vi "Main.vi"() -> ()   [LabVIEW 2021]
doc: "The myRIO Project template acquires acceleration data from the onboard accelerometer and displays the changes of acceleration values in a waveform chart."
uses:
  <vilib>/myRIO/Instrument Drivers/Onboard IO/AI/typedefs/AI Reference.ctl
  <vilib>/myRIO/Common/Instrument Driver Framework/Utilities/typedefs/myRIO Generic Hardware Reference.ctl
  <vilib>/myRIO/Common/Instrument Driver Framework/Utilities/typedefs/Hardware Version Enum.ctl
  <vilib>/myRIO/Common/Instrument Driver Framework/Utilities/typedefs/myRIO v1.0 Reference.ctl
  <vilib>/myRIO/Common/Instrument Driver Framework/Utilities/typedefs/Generic FPGA Reference.ctl
  <vilib>/myRIO/Common/Instrument Driver Framework/myRIO v1.0/AI/typedefs/AI Channels List.ctl
  <vilib>/myRIO/Common/Instrument Driver Framework/myRIO v1.0/AI/typedefs/AI Channels Enum.ctl
  <vilib>/myRIO/Common/Instrument Driver Framework/Utilities/typedefs/Analog Scaling Constants List.ctl
  <vilib>/myRIO/Common/Instrument Driver Framework/Utilities/typedefs/Analog Scaling Constants.ctl
  <vilib>/userDefined/High Color/nirio_resource_hc.ctl
  <vilib>/myRIO/Instrument Drivers/Onboard IO/DIO/typedefs/DIO Reference.ctl
  <vilib>/myRIO/Common/Instrument Driver Framework/myRIO v1.0/DIO/typedefs/DIO Channels List.ctl
  <vilib>/myRIO/Common/Instrument Driver Framework/myRIO v1.0/DIO/typedefs/DIO Channels Enum.ctl
  <vilib>/myRIO/Common/Instrument Driver Framework/myRIO v1.0/AI/vis/myRIO v1.1 Open AI.vi
  <vilib>/myRIO/Common/Instrument Driver Framework/myRIO v1.0/DIO/vis/myRIO v1.1 Open DIO.vi
  <vilib>/myRIO/Common/Instrument Driver Framework/Utilities/vis/Validate Channels.vi
  <vilib>/myRIO/Common/Instrument Driver Framework/myRIO v1.0/AI/vis/myRIO v1.0 Reserve AI.vi
  <vilib>/myRIO/Common/Instrument Driver Framework/myRIO v1.0/DIO/vis/myRIO v1.0 Reserve DIO.vi
  <vilib>/myRIO/Common/Instrument Driver Framework/myRIO v1.0/AI/vis/myRIO v1.0 Close AI.vi
  <vilib>/myRIO/Common/Instrument Driver Framework/myRIO v1.0/DIO/vis/myRIO v1.0 Close DIO.vi
  <vilib>/myRIO/Common/Instrument Driver Framework/myRIO v1.0/AI/vis/myRIO v1.0 Build MUX Configuration AI.vi
  <vilib>/myRIO/Common/Instrument Driver Framework/myRIO v1.0/Resource Manager/vis/myRIO v1.0 Reserve Channel List.vi
  <vilib>/myRIO/Common/Instrument Driver Framework/myRIO v1.0/DIO/vis/myRIO v1.0 Build MUX Configuration DIO.vi
  <vilib>/myRIO/Common/Instrument Driver Framework/myRIO v1.0/AI/vis/myRIO v1.0 Unreserve AI.vi
  <vilib>/myRIO/Common/Instrument Driver Framework/myRIO v1.0/DIO/vis/myRIO v1.0 Unreserve DIO.vi
  <vilib>/myRIO/Common/Instrument Driver Framework/myRIO v1.0/Resource Manager/vis/myRIO v1.0 Reserve Channel.vi
  <vilib>/myRIO/Common/Instrument Driver Framework/myRIO v1.0/Resource Manager/vis/myRIO v1.0 Unreserve Channel.vi
  <vilib>/myRIO/Common/Instrument Driver Framework/myRIO v1.0/Resource Manager/vis/myRIO v1.0 Create Configuration List.vi
  <vilib>/myRIO/Common/Instrument Driver Framework/myRIO v1.0/Resource Manager/vis/myRIO v1.0 Unreserve Channel List.vi
  <vilib>/myRIO/Common/Instrument Driver Framework/myRIO v1.0/Resource Manager/vis/myRIO v1.0 Build Mutex Name.vi
  <vilib>/Utility/VariantDataType/GetNumericInfo.vi
  <vilib>/Utility/error.llb/Error Cluster From Error Code.vi
  <vilib>/myRIO/Common/Instrument Driver Framework/myRIO v1.0/myRIO v1.1 Open.vi
  <vilib>/myRIO/Common/Instrument Driver Framework/Utilities/vis/IO Manager.vi
  <vilib>/myRIO/Common/Instrument Driver Framework/Utilities/vis/Configuration Manager.vi
  <vilib>/myRIO/Common/Instrument Driver Framework/myRIO v1.0/Resource Manager/vis/myRIO v1.0 Configure IO.vi
  <vilib>/myRIO/Common/Instrument Driver Framework/myRIO v1.0/myRIO v1.0 Close.vi
  <vilib>/myRIO/Common/Instrument Driver Framework/myRIO v1.0/AI/vis/myRIO v1.0 Get Scaling Constants AI.vi
  <vilib>/myRIO/Common/Instrument Driver Framework/myRIO v1.0/AI/vis/myRIO v1.0 Read AI.vi
  <vilib>/myRIO/Common/Instrument Driver Framework/myRIO v1.0/DIO/vis/myRIO v1.0 Read DIO.vi
  <vilib>/myRIO/Common/Instrument Driver Framework/myRIO v1.0/DIO/vis/myRIO v1.0 Write DIO.vi
  <vilib>/myRIO/Common/Instrument Driver Framework/myRIO v1.0/DIO/vis/myRIO v1.0 Shutdown DIO.vi
  <vilib>/myRIO/Instrument Drivers/Onboard IO/DIO/vis/myRIO DIO Open.xnode
  <vilib>/myRIO/Instrument Drivers/Onboard IO/AI/vis/myRIO AI Open.xnode
  <vilib>/myRIO/Instrument Drivers/Onboard IO/DIO/DIO.lvlib
  <vilib>/myRIO/Instrument Drivers/Onboard IO/AI/AI.lvlib
panel:
  out "A/AI0 (Pin 3)":dbl
  in  "Stop Button":bool
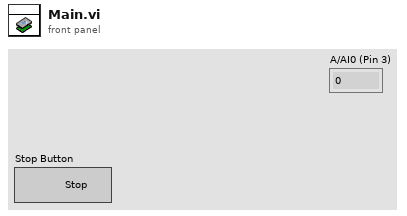
[diagram p1: front panel]
types:
  T1 = typedef "AI.lvlib/AI Reference.ctl" = cluster{"myRIO Reference":T2, "AI Channels List":T6, "AI Scaling Constants List":T8}
  T2 = typedef "myRIO Generic Hardware Reference.ctl" = cluster{"myRIO Model":T3, "myRIO Hardware Reference":T4}
  T3 = typedef "Hardware Version Enum.ctl" = enum16{"Unknown", "myRIO-1900", "myRIO-1950", "roboRIO", "NI ELVIS RIO CM", "ELVIS III"}
  T4 = typedef "myRIO v1.0 Reference.ctl" = cluster{"Generic FPGA Reference":T5, "Allow multiple opens":bool}
  T5 = typedef "Generic FPGA Reference.ctl" = refnum<k20>
  T6 = typedef "AI Channels List.ctl" = T7[]
  T7 = typedef "AI Channels Enum.ctl" = enum16{"Not Connected", "AudioIn/Left", "AudioIn/Right", "C/AI0", "C/AI1", "A/AI0", "A/AI1", "A/AI2", "A/AI3", "A/AI4", "A/AI5", "A/AI6", "A/AI7", "B/AI0", "B/AI1", "B/AI2", "B/AI3", "B/AI4", "B/AI5", "B/AI6", "B/AI7", "AI/AI0", "AI/AI1", "AI/AI2", "AI/AI3", "A/AI0 (DIFF)", "A/AI1 (DIFF)", "A/AI2 (DIFF)", "A/AI3 (DIFF)", "B/AI0 (DIFF)", "B/AI1 (DIFF)", "B/AI2 (DIFF)", "B/AI3 (DIFF)"}
  T8 = typedef "Analog Scaling Constants List.ctl" = T9[]
  T9 = typedef "Analog Scaling Constants.ctl" = cluster{"LSB Weight (Volts)":dbl, "Offset (Volts)":dbl, "Signed?":bool}
  T10 = typedef "DIO.lvlib/DIO Reference.ctl" = cluster{"myRIO Reference":T2, "DIO Channels List":T11}
  T11 = typedef "DIO Channels List.ctl" = T12[]
  T12 = typedef "DIO Channels Enum.ctl" = enum16{"Not Connected", "C/DIO0", "C/DIO1", "C/DIO2", "C/DIO3", "C/DIO4", "C/DIO5", "C/DIO6", "C/DIO7", "A/DIO0", "A/DIO1", "A/DIO2", "A/DIO3", "A/DIO4", "A/DIO5", "A/DIO6", "A/DIO7", "A/DIO8", "A/DIO9", "A/DIO10", "A/DIO11", "A/DIO12", "A/DIO13", "A/DIO14", "A/DIO15", "A/DIO16", "A/DIO17", "A/DIO18", "A/DIO19", "B/DIO0", "B/DIO1", "B/DIO2", "B/DIO3", "B/DIO4", "B/DIO5", "B/DIO6", "B/DIO7", "B/DIO8", "B/DIO9", "B/DIO10", "B/DIO11", "B/DIO12", "B/DIO13", "B/DIO14", "B/DIO15", "B/DIO16", "B/DIO17", "B/DIO18", "B/DIO19", "LED0", "LED1", "LED2", "LED3", "Button0", "DIO/DIO0", "DIO/DIO1", "DIO/DIO2", "DIO/DIO3", "DIO/DIO4", "DIO/DIO5", "DIO/DIO6", "DIO/DIO7", "DIO/DIO8", "DIO/DIO9", "SPI/CS0", "SPI/CS1", "SPI/CS2", "SPI/CS3", "LED RADIO (Green)", "LED RADIO (Red)", "LED COMM (Green)", "LED COMM (Red)", "LED MODE (Green)", "LED MODE (Red)"}
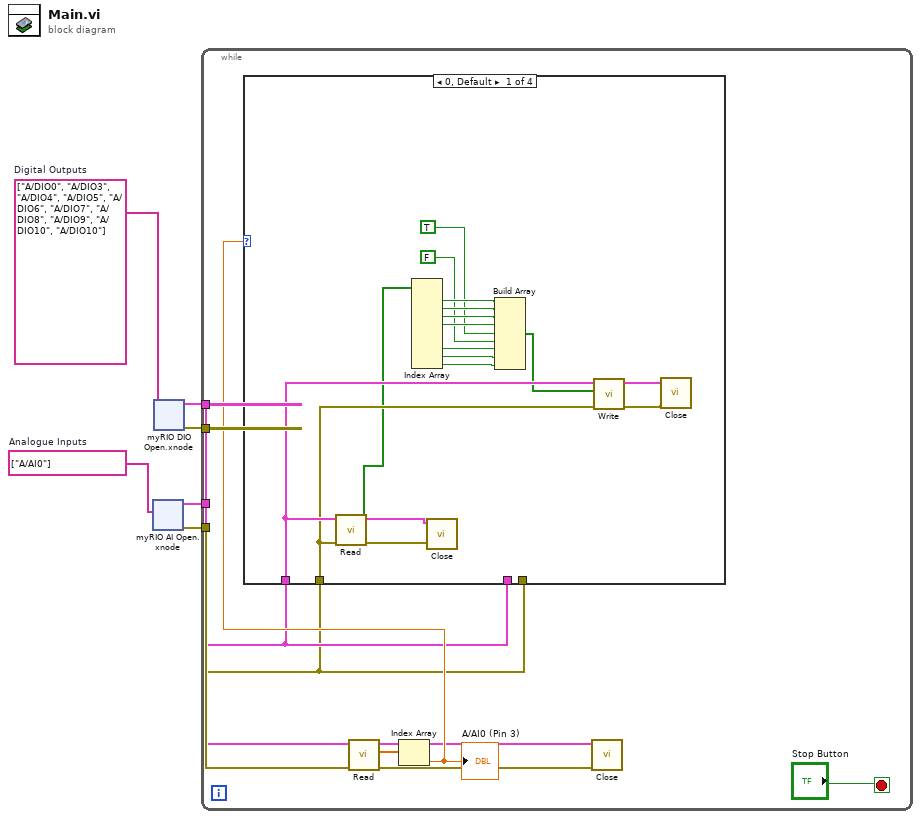
[diagram p0: block diagram]
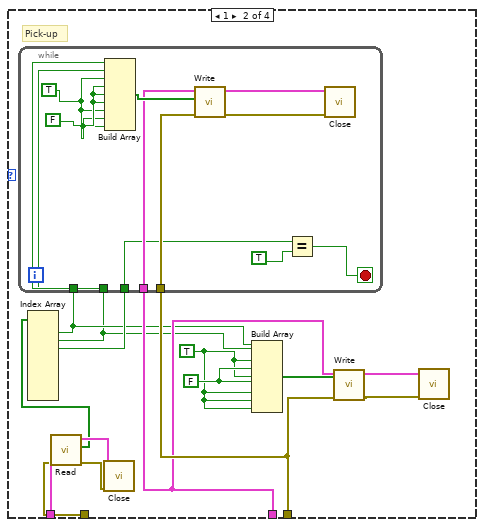
[diagram p2: hidden frame]
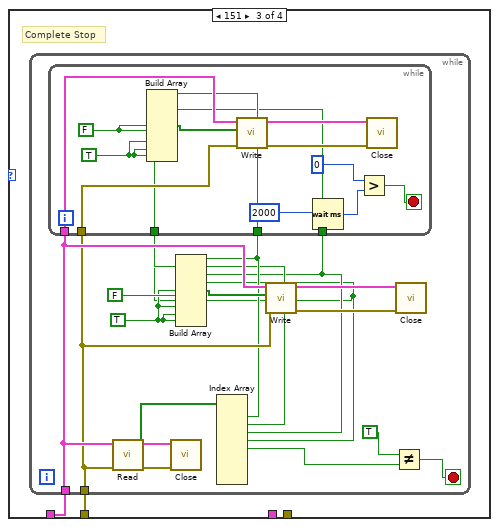
[diagram p3: hidden frame]
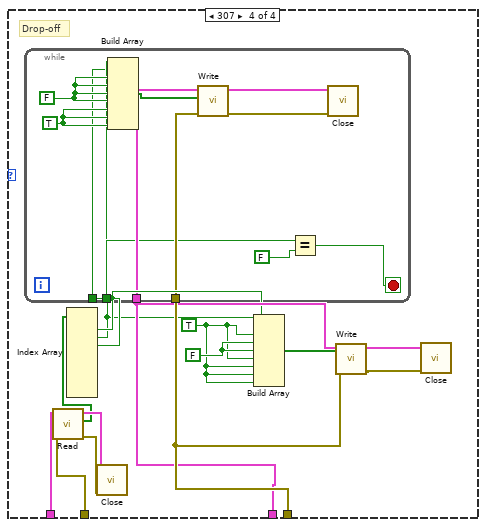
[diagram p4: hidden frame]
diagram:
  w3 = tag[] ["A/AI0"]  # Analogue Inputs
  w4 = tag[] ["A/DIO0", "A/DIO3", "A/DIO4", "A/DIO5", "A/DIO6", "A/DIO7", "A/DIO8", "A/DIO9", "A/DIO10", "A/DIO10"]  # Digital Outputs
  n1 = xnode "myRIO AI Open.xnode"("Channel Names"=w3) -> ("error out"=w2:errorcluster, "AI Ref Out"=w1:T1)  [unwired: 2 in]
  n2 = xnode "myRIO DIO Open.xnode"("Channel Names"=w4) -> ("error out"=w5:errorcluster, "DIO Ref Out"=w6:T10)  [unwired: 2 in]
  n3 = while {
    tunnel: w6 -> [w10]
    tunnel: w5 -> [w9]
    tunnel: w2 -> [w14]
    tunnel: w1 -> [w13]
    stop <- "Stop Button" stop-if-true
    n4 = call <vilib>:"Read.vi"("error in (no error)"=w14, "AI Ref In"=w13) -> ("error out"=w7:errorcluster, "Values"=w12:dbl[], "AI Ref Out"=w8:T1)  [unwired: 7 in]
    n5 = Index Array(array=w12) -> (element=w11:dbl)  [unwired: 1 in]
    "A/AI0 (Pin 3)" <- w11
    n6 = case shown="0, Default" w11 {
      tunnel: w10 -> [_ w42 _ w102]
      tunnel: w9 -> [_ w43 _ w103]
      tunnel: w10 -> [w32 w47 w61 w105]
      tunnel: w9 -> [w31 w46 w60 w104]
      frame 0, Default {
        n7 = call <vilib>:"Read.vi"("error in (no error)"=w31, "DIO Ref In"=w32) -> ("error out"=w18:errorcluster, "Values"=w29:bool[], "DIO Ref Out"=w19:T10)  [unwired: 7 in]
        n8 = Index Array(array=w29) -> (element #1=w28:bool, element #2=w27:bool, element #3=w26:bool, element #4=w25:bool, element #7=w24:bool, element #8=w23:bool, element #9=w22:bool)  [unwired: 9 in, 2 out]
        n9 = call <vilib>:"Close.vi"("error in (no error)"=w18, "DIO Ref In"=w19) -> ()  [unwired: 9 in, 1 out]
        n10 = Build Array(w28, w27, w26, w25, TRUE, FALSE, w24, w23, w22) -> (w30:bool[])
        n11 = call <vilib>:"Write.vi"("error in (no error)"=w31, "Values"=w30, "DIO Ref In"=w32) -> ("error out"=w20:errorcluster, "DIO Ref Out"=w21:T10)  [unwired: 6 in]
        n12 = call <vilib>:"Close.vi"("error in (no error)"=w20, "DIO Ref In"=w21) -> ()  [unwired: 9 in, 1 out]
      }
      frame 1 {
        w41 = TRUE
        w45 = FALSE
        # "Pick-up"
        n13 = call <vilib>:"Read.vi"("error in (no error)"=w46, "DIO Ref In"=w47) -> ("error out"=w37:errorcluster, "Values"=w36:bool[], "DIO Ref Out"=w38:T10)  [unwired: 7 in]
        n14 = Index Array(array=w36) -> (element #1=w34:bool, element #2=w33:bool, element #3=w35:bool)  [unwired: 9 in, 6 out]
        n15 = while {
          tunnel: w42 -> [w56]
          tunnel: w43 -> [w55]
          tunnel: w35 -> [w50]
          tunnel: w34 -> [w49]
          tunnel: w33 -> [w48]
          stop <- w54 stop-if-true
          w58 = TRUE
          w59 = FALSE
          n16 = Build Array(w49, w48, w58, w59, w59, w59, w58, w58, w58) -> (w57:bool[])
          n17 = call <vilib>:"Write.vi"("error in (no error)"=w55, "Values"=w57, "DIO Ref In"=w56) -> ("error out"=w51:errorcluster, "DIO Ref Out"=w52:T10)  [unwired: 6 in]
          n18 = Equal?(x=w50, y=TRUE) -> (x = y?=w54:bool)
          n19 = call <vilib>:"Close.vi"("error in (no error)"=w51, "DIO Ref In"=w52) -> ()  [unwired: 9 in, 1 out]
        }
        n20 = call <vilib>:"Close.vi"("error in (no error)"=w37, "DIO Ref In"=w38) -> ()  [unwired: 9 in, 1 out]
        n21 = Build Array(w34, w33, w41, w45, w41, w45, w41, w41, w41) -> (w44:bool[])
        n22 = call <vilib>:"Write.vi"("error in (no error)"=w43, "Values"=w44, "DIO Ref In"=w42) -> ("error out"=w39:errorcluster, "DIO Ref Out"=w40:T10)  [unwired: 6 in]
        n23 = call <vilib>:"Close.vi"("error in (no error)"=w39, "DIO Ref In"=w40) -> ()  [unwired: 9 in, 1 out]
      }
      frame 151 {
        # "Complete Stop"
        n24 = while {
          tunnel: w61 -> [w68]
          tunnel: w60 -> [w67]
          stop <- w78 stop-if-true
          w66 = TRUE
          n25 = call <vilib>:"Read.vi"("error in (no error)"=w67, "DIO Ref In"=w68) -> ("error out"=w76:errorcluster, "Values"=w74:bool[], "DIO Ref Out"=w75:T10)  [unwired: 7 in]
          n26 = call <vilib>:"Close.vi"("error in (no error)"=w76, "DIO Ref In"=w75) -> ()  [unwired: 9 in, 1 out]
          n27 = Index Array(array=w74) -> (element #1=w65:bool, element #2=w64:bool, element #3=w63:bool, element #4=w62:bool, element #5=w73:bool)  [unwired: 9 in, 4 out]
          n28 = while {
            tunnel: w68 -> [w88]
            tunnel: w67 -> [w87]
            tunnel: w65 -> [w82]
            tunnel: w64 -> [w81]
            tunnel: w63 -> [w80]
            tunnel: w62 -> [w79]
            stop <- w84 stop-if-true
            w89 = TRUE
            w90 = FALSE
            n29 = Build Array(w82, w81, w80, w79, w90, w90, w89, w89, w89) -> (w93:bool[])
            n30 = call <vilib>:"Write.vi"("error in (no error)"=w87, "Values"=w93, "DIO Ref In"=w88) -> ("error out"=w91:errorcluster, "DIO Ref Out"=w92:T10)  [unwired: 6 in]
            n31 = Wait (ms)(milliseconds to wait=2000) -> (millisecond timer value=w85:u32)
            n32 = Greater?(x=0, y=w85) -> (0:w84:bool)
            n33 = call <vilib>:"Close.vi"("error in (no error)"=w91, "DIO Ref In"=w92) -> ()  [unwired: 9 in, 1 out]
          }
          n34 = Build Array(w65, w64, w63, w62, w66, FALSE, w66, w66, w66) -> (w72:bool[])
          n35 = call <vilib>:"Write.vi"("error in (no error)"=w67, "Values"=w72, "DIO Ref In"=w68) -> ("error out"=w70:errorcluster, "DIO Ref Out"=w71:T10)  [unwired: 6 in]
          n36 = Not Equal?(x=TRUE, y=w73) -> (x != y?=w78:bool)
          n37 = call <vilib>:"Close.vi"("error in (no error)"=w70, "DIO Ref In"=w71) -> ()  [unwired: 9 in, 1 out]
        }
      }
      frame 307 {
        w98 = TRUE
        w99 = FALSE
        # "Drop-off"
        n38 = call <vilib>:"Read.vi"("error in (no error)"=w104, "DIO Ref In"=w105) -> ("error out"=w100:errorcluster, "Values"=w97:bool[], "DIO Ref Out"=w101:T10)  [unwired: 7 in]
        n39 = Index Array(array=w97) -> (element #1=w95:bool, element #2=w94:bool, element #3=w96:bool)  [unwired: 9 in, 6 out]
        n40 = while {
          tunnel: w103 -> [w115]
          tunnel: w102 -> [w114]
          tunnel: w96 -> [w111]
          tunnel: w95 -> [w110]
          tunnel: w94 -> [w109]
          stop <- w113 stop-if-true
          w117 = TRUE
          w112 = FALSE
          n41 = Build Array(w110, w109, w112, w112, w112, w112, w117, w117, w117) -> (w118:bool[])
          n42 = call <vilib>:"Write.vi"("error in (no error)"=w115, "Values"=w118, "DIO Ref In"=w114) -> ("error out"=w120:errorcluster, "DIO Ref Out"=w119:T10)  [unwired: 6 in]
          n43 = Equal?(x=w111, y=FALSE) -> (x = y?=w113:bool)
          n44 = call <vilib>:"Close.vi"("error in (no error)"=w120, "DIO Ref In"=w119) -> ()  [unwired: 9 in, 1 out]
        }
        n45 = call <vilib>:"Close.vi"("error in (no error)"=w100, "DIO Ref In"=w101) -> ()  [unwired: 9 in, 1 out]
        n46 = Build Array(w95, w94, w98, w99, w99, w98, w98, w98, w98) -> (w106:bool[])
        n47 = call <vilib>:"Write.vi"("error in (no error)"=w103, "Values"=w106, "DIO Ref In"=w102) -> ("error out"=w108:errorcluster, "DIO Ref Out"=w107:T10)  [unwired: 6 in]
        n48 = call <vilib>:"Close.vi"("error in (no error)"=w108, "DIO Ref In"=w107) -> ()  [unwired: 9 in, 1 out]
      }
    }
    n49 = call <vilib>:"Close.vi"("error in (no error)"=w7, "AI Ref In"=w8) -> ()  [unwired: 9 in, 1 out]
  }
